vi "add alarm comparison.vi"(5 "Limit":dbl, 6 "comparison name":string, 7 "comparison":T2, 8 "error in":errorcluster, 9 "data type":T1, 10 "alarm name":string, 11 "alarms module configuration in":refnum<class "tag select module configuration.lvclass">) -> (0 "error out":errorcluster, 1 "created channels":refnum<class "TBM channel.lvclass">[](array[class]), 2 "compare index":i32, 3 "alarms module configuration out":refnum<class "tag select module configuration.lvclass">)   [LabVIEW 2013]
uses:
  tag select module configuration.lvclass
  <vilib>/NI/Tag Bus Module Framework/channel/TBM channel.lvclass
  compare type.ctl
  alarm comparison.ctl
  <vilib>/NI/Configuration Framework/serializable configuration/NISE_CEF_serializable configuration.lvclass
  <vilib>/NI/Tag Bus Module Framework/channel/channel classification.ctl
  <vilib>/NI/Tag Bus/tag/Data Type.ctl
  <vilib>/NI/Tag Bus/tag/tag descriptor.lvclass
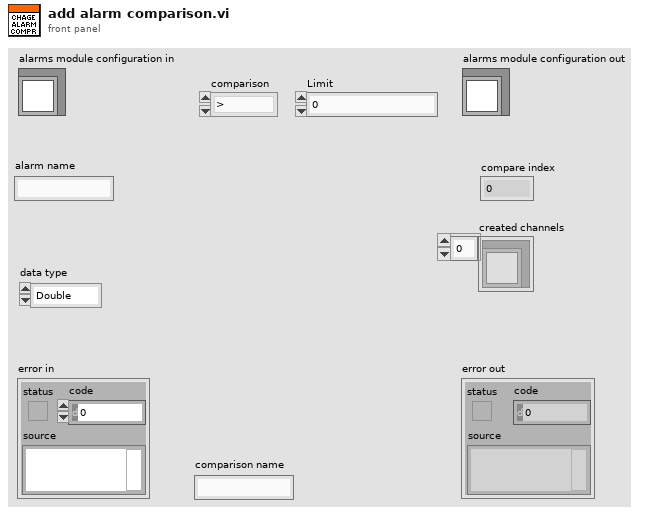
[diagram p1: front panel]
types:
  T1 = typedef "tag bus.lvlib/tag descriptor.lvclass/Data Type.ctl" = enum16{"Double", "Single", "I64", "I32", "I16", "I8", "U64", "U32", "U16", "U8", "Boolean", "String", "Array of Double", "Array of Single", "Array of I64", "Array of I32", "Array of I16", "Array of I8", "Array of U64", "Array of U32", "Array of U16", "Array of U8", "Array of Boolean", "Array of String"}
  T2 = typedef "compare type.ctl" = enum16{">", "<", ">=", "<=", "="}
  T3 = typedef "TBM channel.lvclass/channel classification.ctl" = enum16{"input data", "output data", "processing parameter", "processing result"}
  T4 = typedef "alarm comparison.ctl" = cluster{"input channel":refnum<class "TBM channel.lvclass">, "limit":dbl, "comparison":T2}
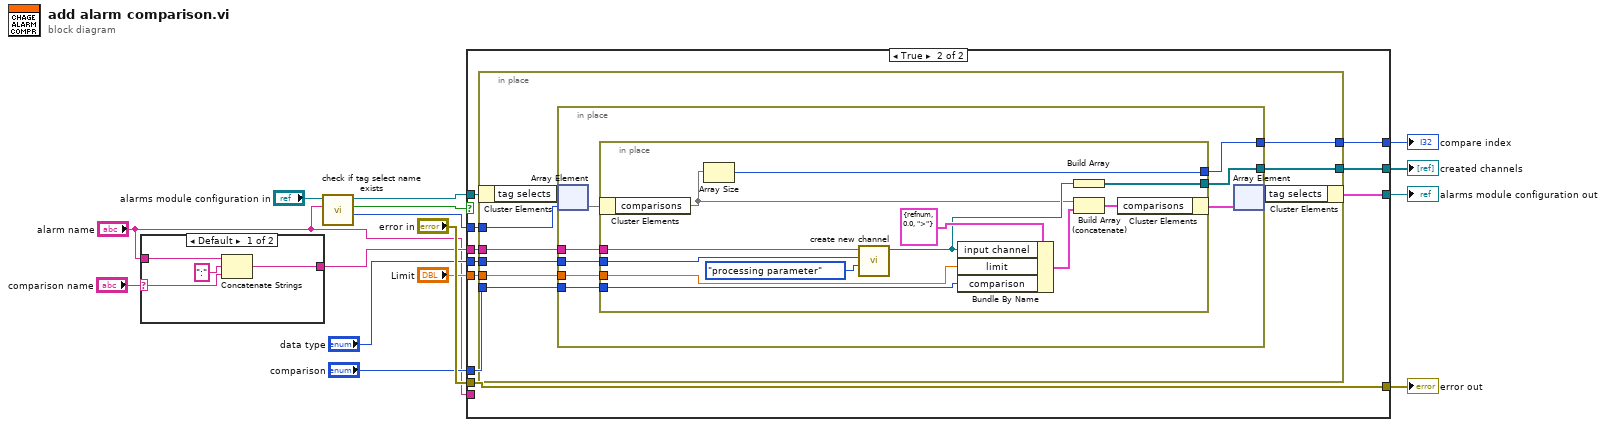
[diagram p0: block diagram]
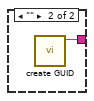
[diagram p2: hidden frame]
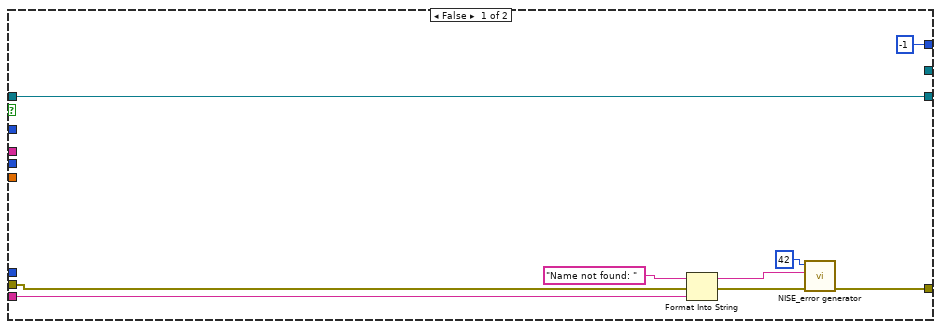
[diagram p3: hidden frame]
diagram:
  n1 = case shown="Default" "comparison name" {
    selector: "comparison name" -> [w19 _]
    tunnel: [w18 w20] -> w2
    tunnel: "alarm name" -> [w17 _]
    frame Default {
      n2 = Concatenate Strings(w17, ":" ("string"), w19) -> (w18:string)
    }
    frame "" {
      n3 = call <vilib>:"create GUID.vi"() -> ("uuid"=w20:string)  [unwired: 10 in, 1 out]
    }
  }
  n4 = call "check if tag select name exists.vi"("name to locate"="alarm name", "tag select module configuration in"="alarms module configuration in") -> ("index"=w9:i32, "found?"=w12:bool, "tag select module configuration out"=w10:refnum<class "tag select module configuration.lvclass">)  [unwired: 6 in, 1 out]
  n5 = case shown="True" w12 {
    tunnel: [w28 w37] -> w14
    tunnel: "error in" -> [w29 w37]
    tunnel: [w23 w38] -> w11
    tunnel: w10 -> [w23 w39]
    tunnel: w9 -> [_ w36]
    tunnel: "alarm name" -> [w22 _]
    tunnel: "Limit" -> [_ w35]
    tunnel: "comparison" -> [_ w34]
    tunnel: "data type" -> [_ w33]
    tunnel: [_ w32] -> w5
    tunnel: [-1 w31] -> w4
    tunnel: w2 -> [_ w30]
    frame False {
      n6 = Format Into String(initial string="Name not found: " ("append error message"), error in=w29, w22) -> (resulting string=w24:string, error out=w26:errorcluster)  [unwired: 1 in]
      n7 = call <vilib>:"NISE_error generator.vi"("error in"=w26, "append error message"=w24, "error code (0)"=42) -> ("error out"=w28:errorcluster)  [unwired: 6 in]
    }
    frame True {
      n8 = in-place {
        in-place-border: w36 -> [w46]
        in-place-border: w35 -> [w45]
        in-place-border: w34 -> [w44]
        in-place-border: w33 -> [w43]
        in-place-border: [w42] -> w32
        in-place-border: [w41] -> w31
        in-place-border: w30 -> [w40]
        n9 = in-place-cluster #1(w39) -> ("tag selects"=w48)
        n10 = in-place {
          in-place-border: w45 -> [w55]
          in-place-border: w44 -> [w54]
          in-place-border: w43 -> [w52]
          in-place-border: [w51] -> w42
          in-place-border: [w50] -> w41
          in-place-border: w40 -> [w49]
          n11 = in-place-array #2(w48, w46) -> (w56)
          n12 = in-place {
            in-place-border: w55 -> [w68]
            in-place-border: w54 -> [w67]
            in-place-border: w52 -> [w62]
            in-place-border: [w60] -> w51
            in-place-border: [w58] -> w50
            in-place-border: w49 -> [w57]
            n13 = in-place-cluster #3(w56) -> ("comparisons"=w59)
            n14 = Array Size(array=w59) -> (size(s)=w58:i32)
            n15 = call <vilib>:"create new channel.vi"("channel classification"=channel_classification."processing parameter", "data type"=w62, "channel name"=w57) -> ("channel"=w61:refnum<class "TBM channel.lvclass">)  [unwired: 8 in]
            n16 = Bundle By Name(cluster=T4 {"input channel"=refnum, "limit"=0.0, "comparison"=enum.">"} ("element"), "input channel"=w61, "limit"=w68, "comparison"=w67) -> (w64:T4)
            n17 = Build Array(w61) -> (w60:refnum<class "TBM channel.lvclass">[])
            n18 = Build Array (concatenate)(w59, w64) -> (w65:T4[])
            n19 = in-place-cluster #3("comparisons"=w65) -> (w53:cluster{})
          }
          n20 = in-place-array #2(w53) -> (w47)  [unwired: 1 out]
        }
        n21 = in-place-cluster #1("tag selects"=w47) -> (w38:cluster{})
      }
    }
  }
  "error out" <- w14
  "alarms module configuration out" <- w11
  "compare index" <- w4
  "created channels" <- w5
